vi "RP-SWITCH CHANNEL.vi"(2 "error in":errorcluster, 3 "Channel":i32, 4 "IP address":string="192.168.4.129") -> (0 "error out":errorcluster, 1 "Switch ok ?":bool)   [LabVIEW 2021]
uses:
  <vilib>/regexp/Match Regular Expression.xnode
  Red_Pitaya_LabVIEW_Driver&Examples/Red_Pitaya/RedPitaya.lvlib
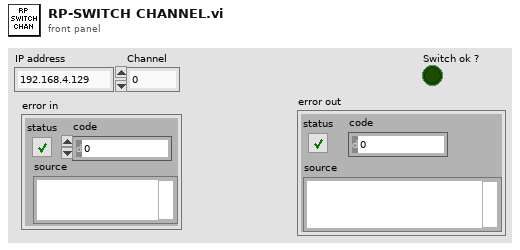
[diagram p1: front panel]
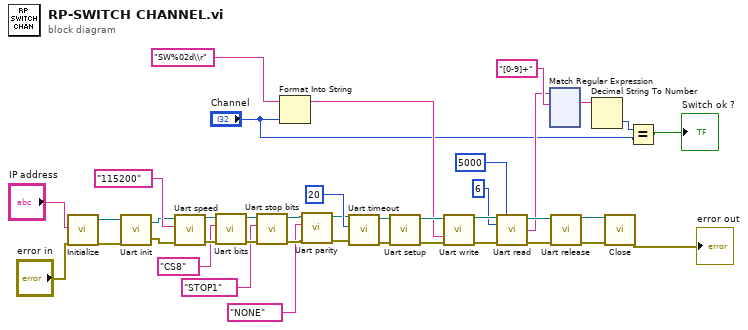
[diagram p0: block diagram]
diagram:
  n1 = call "Initialize.vi"("IP address"="IP address", "error in"="error in") -> ("RedPitaya connection out"=w35:refnum<k5>, "error out"=w34:errorcluster)  [unwired: 16 in]
  n2 = call "Uart init.vi"("error in"=w34, "RedPitaya connection in"=w35) -> ("error out"=w33:errorcluster, "RedPitaya connection out"=w36:refnum<k5>)  [unwired: 2 in]
  n3 = call "Uart speed.vi"("error in"=w33, "speed"="115200" ("Baud Rate (9600)"), "RedPitaya connection in"=w36) -> ("error out"=w4:errorcluster, "RedPitaya connection out"=w5:refnum<k5>)  [unwired: 7 in]
  n4 = call "Uart bits.vi"("error in"=w4, "Bits format"="CS8", "RedPitaya connection in"=w5) -> ("error out"=w6:errorcluster, "RedPitaya connection out"=w7:refnum<k5>)  [unwired: 7 in]
  n5 = call "Uart stop bits.vi"("error in"=w6, "Stop bits"="STOP1", "RedPitaya connection in"=w7) -> ("error out"=w9:errorcluster, "RedPitaya connection out"=w8:refnum<k5>)  [unwired: 7 in]
  n6 = Format Into String(format string="SW%02d\\r", "Channel") -> (resulting string=w21:string)  [unwired: 2 in, 1 out]
  n7 = call "Uart parity.vi"("error in"=w9, "Parity"="NONE", "RedPitaya connection in"=w8) -> ("error out"=w10:errorcluster, "RedPitaya connection out"=w11:refnum<k5>)  [unwired: 7 in]
  n8 = call "Uart timeout.vi"("error in"=w10, "Timeout (*0.1s)"=u8 20, "RedPitaya connection in"=w11) -> ("error out"=w32:errorcluster, "RedPitaya connection out"=w24:refnum<k5>)  [unwired: 7 in]
  n9 = call "Uart setup.vi"("error in"=w32, "RedPitaya connection in"=w24) -> ("error out"=w31:errorcluster, "RedPitaya connection out"=w23:refnum<k5>)  [unwired: 8 in]
  n10 = call "Uart write.vi"("RedPitaya connection in"=w23, "string to send"=w21, "error in"=w31) -> ("RedPitaya connection out"=w25:refnum<k5>, "error out"=w30:errorcluster)  [unwired: 11 in]
  n11 = call "Uart read.vi"("RedPitaya connection in"=w25, "timeout ms (2000)"=5000, "Len"=u8 6, "error in"=w30) -> ("RedPitaya connection out"=w26:refnum<k5>, "Output string"=w19:string, "error out"=w29:errorcluster)  [unwired: 8 in, 1 out]
  n12 = xnode "Match Regular Expression"("input string"=w19, "regular expression"="[0-9]+") -> ("whole match"=w18:string)  [unwired: 4 in, 4 out]
  n13 = call "Uart release.vi"("error in"=w29, "RedPitaya connection in"=w26) -> ("error out"=w28:errorcluster, "RedPitaya connection out"=w27:refnum<k5>)  [unwired: 8 in]
  n14 = Decimal String To Number(string=w18) -> (number=w16:i32)  [unwired: 2 in, 1 out]
  n15 = call "Close.vi"("RedPitaya connection in"=w27, "error in"=w28) -> ("error out"=→"error out":errorcluster)  [unwired: 17 in]
  n16 = Equal?(x=w16, y="Channel") -> (x = y?=→"Switch ok ?":bool)
